vi "enc_a_I16.vi"(1 "Array In":i16[](array[numeric])) -> (0 "Array Out":u8[](array[numeric]))   [LabVIEW 2016, in "MsgPack.lvlib"]
uses:
  MsgPack.lvlib
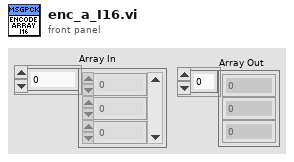
[diagram p1: front panel]
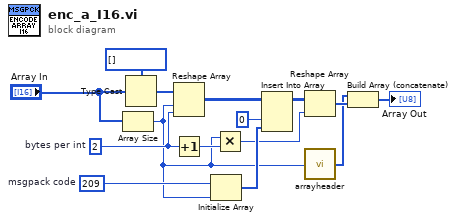
[diagram p0: block diagram]
diagram:
  w11 = u8 209  # msgpack code
  w14 = 2  # bytes per int
  n1 = Array Size(array="Array In") -> (size(s)=w5:i32)
  n2 = Type Cast(type=u8[] [], x="Array In") -> (*(type *) &x=w12:u8[])
  n3 = Reshape Array(w12, w5, w14) -> (w10:u8[][])
  n4 = Increment(x=w14) -> (x+1=w6:i32)
  n5 = Initialize Array(w11, w5) -> (w9:u8[])
  n6 = Multiply(x=w5, y=w6) -> (x*y=w4:i32)
  n7 = Insert Into Array(array=w10, index (col)=0 ("disabled index (col)"), new element=w9) -> (w8:u8[][])  [unwired: 1 in]
  n8 = Reshape Array(w8, w4) -> (w3:u8[])
  n9 = call "arrayheader.vi"("Number of Elements"=w5) -> ("header"=w2:u8[])
  n10 = Build Array (concatenate)(w2, w3) -> (→"Array Out":u8[])
